vi "GlobalCostants.vi"() -> ()   [LabVIEW 2010]
uses:
  VarableStruct.ctl
  VarableID.ctl
panel:
  in  "PortIPList":string[](array[string])
  in  "CommandCodeList":cluster{"CommandCode":string, "VarableID":T1}[](array[cluster])=[{"CommandCode"="68####68110435353433", "VarableID"=enum."current"}, {"CommandCode"="68####68110433343435", "VarableID"=enum."voltage"}, {"CommandCode"="68####68110435383433", "VarableID"=enum."power"}, {"CommandCode"="68####68110435393433", "VarableID"=enum."PF"}]
  in  "VarableList":T2[](array[typedef])
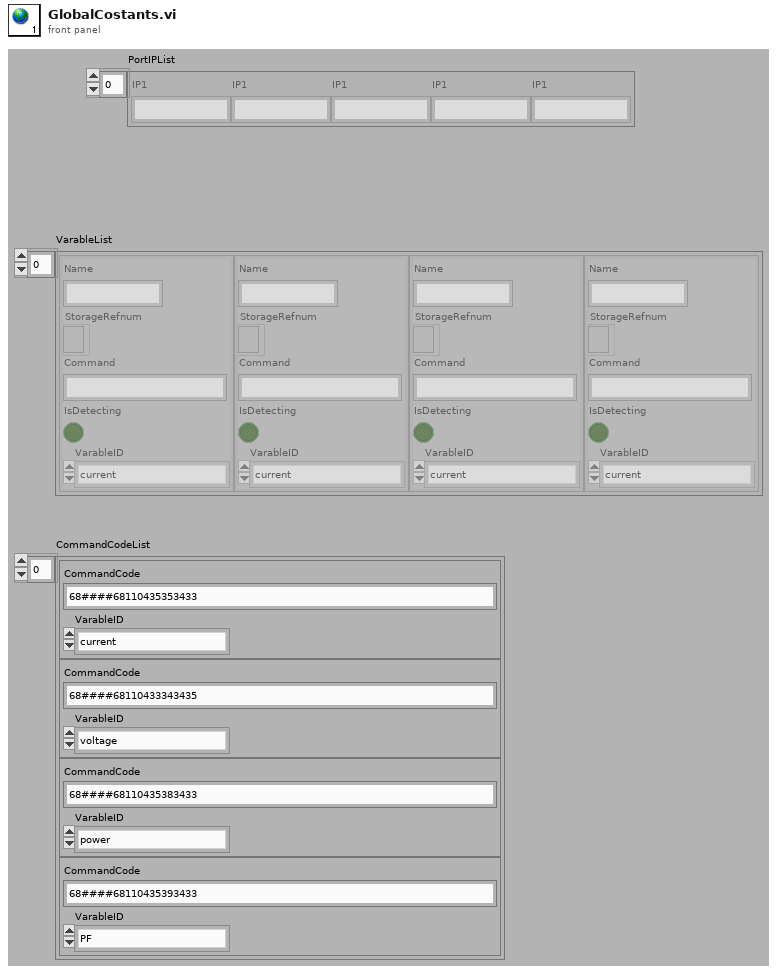
[diagram p1: front panel]
types:
  T1 = typedef "VarableID.ctl" = enum16{"current", "voltage", "power", "PF"}
  T2 = typedef "VarableStruct.ctl" = cluster{"Name":string, "StorageRefnum":refnum<file>, "Command":string, "IsDetecting":bool, "VarableID":T1}
diagram:
